vi "SizeToPicture.vi"(8 "error in (no error)":errorcluster, 10 "Picture Reference":refnum<vi>, 11 "Plot ID":T1 format="%x") -> (0 "error out":errorcluster, 3 "Plot ID Out":T1 format="%x")   [LabVIEW 2013, in "Advanced Plotting Toolkit.lvlib"]
uses:
  Advanced Plotting Toolkit.lvlib
  typedefs/PlotID.ctl
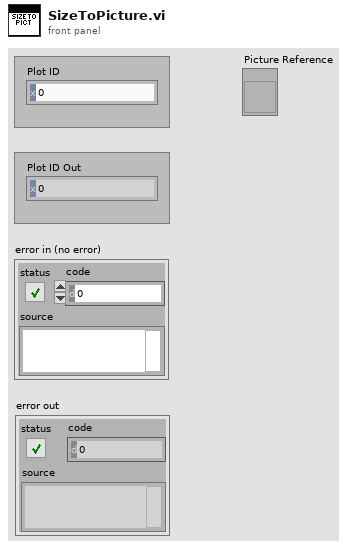
[diagram p1: front panel]
types:
  T1 = typedef "Advanced Plotting Toolkit.lvlib/PlotID.ctl" = i32
  T2 = typedef "LVBoundsTypeDef.ctl" = cluster{"Width":u32, "Height":u32}
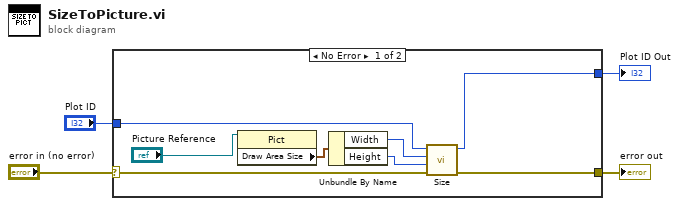
[diagram p0: block diagram]
diagram:
  n1 = case shown="No Error" "error in (no error)" {
    selector: "error in (no error)" -> [w10 w13]
    tunnel: "Plot ID" -> [w11 w14]
    tunnel: [w9 w14] -> w2
    tunnel: [w8 w13] -> w1
    frame No Error {
      n2 = property on="Property Node" class="Pict"(reference="Picture Reference") -> ("Draw Area Size"=w7:T2)  [unwired: 1 in, 2 out]
      n3 = Unbundle By Name(w7) -> ("Width"=w6:u32, "Height"=w5:u32)
      n4 = call "Size.vi"("error in (no error)"=w10, "Height (pixels)"=w5, "Width (pixels)"=w6, "Plot ID"=w11) -> ("error out"=w8:errorcluster, "Plot ID Out"=w9:T1)  [unwired: 6 in]
    }
    frame Error {
    }
  }
  "Plot ID Out" <- w2
  "error out" <- w1
